vi "RampVoltagewithDDSV14.vi"() -> ()   [LabVIEW 2016]
uses:
  <vilib>/DAQmx/write.llb/DAQmx Write (Digital 1D Wfm NChan NSamp).vi
  <vilib>/DAQmx/write.llb/DAQmx Write (Analog 2D DBL NChan NSamp).vi
  <vilib>/DAQmx/create/channels.llb/DAQmx Create Channel (AO-Voltage-Basic).vi
  <vilib>/DAQmx/create/channels.llb/DAQmx Create Channel (DO-Digital Output).vi
  <vilib>/DAQmx/configure/timing.llb/DAQmx Timing (Sample Clock).vi
  <vilib>/DAQmx/configure/trigger.llb/DAQmx Start Trigger (Digital Edge).vi
  <vilib>/Waveform/DWDTOps.llb/DWDT Boolean Array to Digital.vi
  <vilib>/Waveform/DWDTOps.llb/DWDT Uncompress Digital.vi
  <vilib>/DAQmx/miscellaneous.llb/DAQmx Fill In Error Info.vi
  <vilib>/Waveform/DTblOps.llb/DTbl Digital to Analog.vi
  <resource>/objmgr/daqmx.rc
  <vilib>/Utility/file.llb/Write Delimited Spreadsheet (DBL).vi
panel:
  out "ao3 Samples":i32=2001
  out "ao2 Samples":i32=2001
  in  "ao3  File Path":path
  in  "ao2  File Path":path
  in  "Phase Lock Switch\n(TTL High - Lock Off)":bool
  in  "Phase Lock Switch (Port 0 Line 1)":tag="Dev2/port0/line1"
  out "Digital Output":cluster{i32, dbl, dbl[][]}(graph)={0, 1e-05, [[0.0, 0.0, 0.0, 0.0, 0.0, 0.0, 0.0, 0.0, 0.0, 0.0, 0.0, 0.0, 0.0, 0.0, 0.0, 0.0, 0.0, 0.0, 0.0, 0.0, 0.0, 0.0, 0.0, 0.0, 0.0, 0.0, 0.0, 0.0, 0.0, 0.0, 0.0, 0.0, 0.0, 0.0, 0.0, 0.0, 0.0, 0.0, 0.0, 0.0, 0.0, 0.0, 0.0, 0.0, 0.0, 0.0, 0.0, 0.0, 0.0, 0.0, 0.0, 0.0, 0.0, 0.0, 0.0, 0.0, 0.0, 0.0, 0.0, 0.0, 0.0, 0.0, 0.0, 0.0, 0.0, 0.0, 0.0, 0.0, 0.0, 0.0, 0.0, 0.0, 0.0, 0.0, 0.0, 0.0, 0.0, 0.0, 0.0, 0.0, 0.0, 0.0, 0.0, 0.0, 0.0, 0.0, 0.0, 0.0, 0.0, 0.0, 0.0, 0.0, 0.0, 0.0, 0.0, 0.0, 0.0, 0.0, 0.0, 0.0, 0.0, 0.0, 0.0, 0.0, 0.0, 0.0, 0.0, 0.0, 0.0, 0.0, 0.0, 0.0, 0.0, 0.0, 0.0, 0.0, 0.0, 0.0, 0.0, 0.0, 0.0, 0.0, 0.0, 5.0, 5.0, 5.0, 5.0, 5.0, 5.0, 5.0, 5.0, 5.0, 5.0, 5.0, 5.0, 5.0, 5.0, 5.0, 5.0, 5.0, 5.0, 5.0, 5.0, 5.0, 5.0, 5.0, 5.0, 5.0, 5.0, 5.0, 5.0, 5.0, 5.0, 5.0, 5.0, 5.0, 5.0, 5.0, 5.0, 5.0, 5.0, 5.0, 5.0, 5.0, 5.0, 5.0, 5.0, 5.0, 5.0, 5.0, 5.0, 5.0, 5.0, 5.0, 5.0, 5.0, 5.0, 5.0, 5.0, 5.0, 5.0, 5.0, 5.0, 5.0, 5.0, 5.0, 5.0, 5.0, 5.0, 5.0, 5.0, 5.0, 5.0, 5.0, 5.0, 5.0, 5.0, 5.0, 5.0, 5.0, 5.0, 5.0, 5.0, 5.0, 5.0, 5.0, 5.0, 5.0, 5.0, 5.0, 5.0, 5.0, 5.0, 5.0, 5.0, 5.0, 5.0, 5.0, 5.0, 5.0, 5.0, 5.0, 5.0, 5.0, 5.0, 5.0, 5.0, 5.0, 5.0, 5.0, 5.0, 5.0, 5.0, 5.0, 5.0, 5.0, 5.0, 5.0, 5.0, 5.0, 5.0, 5.0, 5.0, 5.0, 5.0, 5.0, 5.0, 5.0, 5.0, 5.0, 5.0, 5.0, 5.0, 5.0, 5.0, 5.0, 5.0, 5.0, 5.0, 5.0, 5.0, 5.0, 5.0, 5.0, 5.0, 5.0, 5.0, 5.0, 5.0, 5.0, 5.0, 5.0, 5.0, 5.0, 5.0, 5.0, 5.0, 5.0, 5.0, 5.0, 5.0, 5.0, 5.0, 5.0, 5.0, 5.0, 5.0, 5.0, 5.0, 5.0, 5.0, 5.0, 5.0, 5.0, 5.0, 5.0, 5.0, 5.0, 5.0, 5.0, 5.0, 5.0, 5.0, 5.0, 5.0, 5.0, 5.0, 5.0, 5.0, 5.0, 5.0, 5.0, 5.0, 5.0, 5.0, 5.0, 5.0, 5.0, 5.0, 5.0, 5.0, 5.0, 5.0, 5.0, 5.0, 5.0, 5.0, 5.0, 5.0, 5.0, 5.0, 5.0, 5.0, 5.0, 5.0, 5.0, 5.0, 5.0, 5.0, 5.0, 5.0, 5.0, 5.0, 5.0, 5.0, 5.0, 5.0, 5.0, 5.0, 5.0, 5.0, 5.0, 5.0, 5.0, 5.0, 5.0, 5.0, 5.0, 5.0, 5.0, 5.0, 5.0, 5.0, 5.0, 5.0, 5.0, 5.0, 5.0, 5.0, 5.0, 5.0, 5.0, 5.0, 5.0, 5.0, 5.0, 5.0, 5.0, 5.0, 5.0, 5.0, 5.0, 5.0, 5.0, 5.0, 5.0, 5.0, 5.0, 5.0, 5.0, 5.0, 5.0, 5.0, 5.0, 5.0, 5.0, 5.0, 5.0, 5.0, 5.0, 5.0, 5.0, 5.0, 5.0, 5.0, 5.0, 5.0, 5.0, 5.0, 5.0, 5.0, 5.0, 5.0, 5.0, 5.0, 5.0, 5.0, 5.0, 5.0, 5.0, 5.0, 5.0, 5.0, 5.0, 5.0, 5.0, 5.0, 5.0, 5.0, 5.0, 5.0, 5.0, 5.0, 5.0, 5.0, 5.0, 5.0, 5.0, 5.0, 5.0, 5.0, 5.0, 5.0, 5.0, 5.0, 5.0, 5.0, 5.0, 5.0, 5.0, 5.0, 5.0, 5.0, 5.0, 5.0, 5.0, 5.0, 5.0, 5.0, 5.0, 5.0, 5.0, 5.0, 5.0, 5.0, 5.0, 5.0, 5.0, 5.0, 5.0, 5.0, 5.0, 5.0, 5.0, 5.0, 5.0, 5.0, 5.0, 5.0, 5.0, 5.0, 5.0, 5.0, 5.0, 5.0, 5.0, 5.0, 5.0, 5.0, 5.0, 5.0, 5.0, 5.0, 5.0, 5.0, 5.0, 5.0, 5.0, 5.0, 5.0, 5.0, 5.0, 5.0, 5.0, 5.0, 5.0, 5.0, 5.0, 5.0, 5.0, 5.0, 5.0, 5.0, 5.0, 5.0, 5.0, 5.0, 5.0, 5.0, 5.0, 5.0, 5.0, 5.0, 0.0, 0.0, 0.0, 0.0, 0.0, 0.0, 0.0, 0.0, 0.0, 0.0, 0.0, 0.0, 0.0, 0.0, 0.0, 0.0, 0.0, 0.0, 0.0, 0.0, 0.0, 0.0, 0.0, 0.0, 0.0, 0.0, 0.0, 0.0, 0.0, 0.0, 0.0, 0.0, 0.0, 0.0, 0.0, 0.0, 0.0, 0.0, 0.0, 0.0, 0.0, 0.0, 0.0, 0.0, 0.0, 0.0, 0.0, 0.0, 0.0, 0.0, 0.0, 0.0, 0.0, 0.0, 0.0, 0.0, 0.0, 0.0, 0.0, 0.0, 0.0, 0.0, 0.0, 0.0, 0.0, 0.0, 0.0, 0.0, 0.0, 0.0, 0.0, 0.0, 0.0, 0.0, 0.0, 0.0, 0.0, 0.0, 0.0, 0.0, 0.0, 0.0, 0.0, 0.0, 0.0, 0.0, 0.0, 0.0, 0.0, 0.0, 0.0, 0.0, 0.0, 0.0, 0.0, 0.0, 0.0, 0.0, 0.0, 0.0, 0.0, 0.0, 0.0, 0.0, 0.0, 0.0, 0.0, 0.0, 0.0, 0.0, 0.0, 0.0, 0.0, 0.0, 0.0, 0.0, 0.0, 0.0, 0.0, 0.0, 0.0, 0.0, 0.0, 0.0, 0.0, 0.0, 0.0, 0.0, 0.0, 0.0, 0.0, 0.0, 0.0, 0.0, 0.0, 0.0, 0.0, 0.0, 0.0, 0.0, 0.0, 0.0, 0.0, 0.0, 0.0, 0.0, 0.0, 0.0, 0.0, 0.0, 0.0, 0.0, 0.0, 0.0, 0.0, 0.0, 0.0, 0.0, 0.0, 0.0, 0.0, 0.0, 0.0, 0.0, 0.0, 0.0, 0.0, 0.0, 0.0, 0.0, 0.0, 0.0, 0.0, 0.0, 0.0, 0.0, 0.0, 0.0, 0.0, 0.0, 0.0, 0.0, 0.0, 0.0, 0.0, 0.0, 0.0, 0.0, 0.0, 0.0, 0.0, 0.0, 0.0, 0.0, 0.0, 0.0, 0.0, 0.0, 0.0, 0.0, 0.0, 0.0, 0.0, 0.0, 0.0, 0.0, 0.0, 0.0, 0.0, 0.0, 0.0, 0.0, 0.0, 0.0, 0.0, 0.0, 0.0, 0.0, 0.0, 0.0, 0.0, 0.0, 0.0, 0.0, 0.0, 0.0, 0.0, 0.0, 0.0, 0.0, 0.0, 0.0, 0.0, 0.0, 0.0, 0.0, 0.0, 0.0, 0.0, 0.0, 0.0, 0.0, 0.0, 0.0, 0.0, 0.0, 0.0, 0.0, 0.0, 0.0, 0.0, 0.0, 0.0, 0.0, 0.0, 0.0, 0.0, 0.0, 0.0, 0.0, 0.0, 0.0, 0.0, 0.0, 0.0, 0.0, 0.0, 0.0, 0.0, 0.0, 0.0, 0.0, 0.0, 0.0, 0.0, 0.0, 0.0, 0.0], [0.0, 0.0, 0.0, 0.0, 0.0, 0.0, 0.0, 0.0, 0.0, 0.0, 0.0, 0.0, 0.0, 0.0, 0.0, 0.0, 0.0, 0.0, 0.0, 0.0, 0.0, 0.0, 0.0, 0.0, 0.0, 0.0, 0.0, 0.0, 0.0, 0.0, 0.0, 0.0, 0.0, 0.0, 0.0, 0.0, 0.0, 0.0, 0.0, 0.0, 0.0, 0.0, 0.0, 0.0, 0.0, 0.0, 0.0, 0.0, 0.0, 0.0, 0.0, 0.0, 0.0, 0.0, 0.0, 0.0, 0.0, 0.0, 0.0, 0.0, 0.0, 0.0, 0.0, 0.0, 0.0, 0.0, 0.0, 0.0, 0.0, 0.0, 0.0, 0.0, 0.0, 0.0, 0.0, 0.0, 0.0, 0.0, 0.0, 0.0, 0.0, 0.0, 0.0, 0.0, 0.0, 0.0, 0.0, 0.0, 0.0, 0.0, 0.0, 0.0, 0.0, 0.0, 0.0, 0.0, 0.0, 0.0, 0.0, 0.0, 0.0, 0.0, 0.0, 0.0, 0.0, 0.0, 0.0, 0.0, 0.0, 0.0, 0.0, 0.0, 0.0, 0.0, 0.0, 0.0, 0.0, 0.0, 0.0, 0.0, 0.0, 0.0, 0.0, 0.0, 0.0, 0.0, 0.0, 0.0, 0.0, 0.0, 0.0, 0.0, 0.0, 0.0, 0.0, 0.0, 0.0, 0.0, 0.0, 0.0, 0.0, 0.0, 0.0, 0.0, 0.0, 0.0, 0.0, 0.0, 0.0, 0.0, 0.0, 0.0, 0.0, 0.0, 0.0, 0.0, 0.0, 0.0, 0.0, 0.0, 0.0, 0.0, 0.0, 0.0, 0.0, 0.0, 0.0, 0.0, 0.0, 0.0, 0.0, 0.0, 0.0, 0.0, 0.0, 0.0, 0.0, 0.0, 0.0, 0.0, 0.0, 0.0, 0.0, 0.0, 0.0, 0.0, 0.0, 0.0, 0.0, 0.0, 0.0, 0.0, 0.0, 0.0, 0.0, 0.0, 0.0, 0.0, 0.0, 0.0, 0.0, 0.0, 0.0, 0.0, 0.0, 0.0, 0.0, 0.0, 0.0, 0.0, 0.0, 0.0, 0.0, 0.0, 0.0, 0.0, 0.0, 0.0, 0.0, 0.0, 0.0, 0.0, 0.0, 0.0, 0.0, 0.0, 0.0, 0.0, 0.0, 0.0, 0.0, 0.0, 0.0, 0.0, 0.0, 0.0, 0.0, 0.0, 0.0, 0.0, 0.0, 0.0, 0.0, 0.0, 0.0, 0.0, 0.0, 0.0, 0.0, 0.0, 0.0, 0.0, 0.0, 0.0, 0.0, 0.0, 0.0, 0.0, 0.0, 0.0, 0.0, 0.0, 0.0, 0.0, 0.0, 0.0, 0.0, 0.0, 0.0, 0.0, 0.0, 0.0, 0.0, 0.0, 0.0, 0.0, 0.0, 0.0, 0.0, 0.0, 0.0, 0.0, 0.0, 0.0, 0.0, 0.0, 0.0, 0.0, 0.0, 0.0, 0.0, 0.0, 0.0, 0.0, 0.0, 0.0, 0.0, 0.0, 0.0, 0.0, 0.0, 0.0, 0.0, 0.0, 0.0, 0.0, 0.0, 0.0, 0.0, 0.0, 0.0, 0.0, 0.0, 0.0, 0.0, 0.0, 0.0, 0.0, 0.0, 0.0, 0.0, 0.0, 0.0, 0.0, 0.0, 0.0, 0.0, 0.0, 0.0, 0.0, 0.0, 0.0, 0.0, 0.0, 0.0, 0.0, 0.0, 0.0, 0.0, 0.0, 0.0, 0.0, 0.0, 0.0, 0.0, 0.0, 0.0, 0.0, 0.0, 0.0, 0.0, 0.0, 0.0, 0.0, 0.0, 0.0, 0.0, 0.0, 0.0, 0.0, 0.0, 0.0, 0.0, 0.0, 0.0, 0.0, 0.0, 0.0, 0.0, 0.0, 0.0, 0.0, 0.0, 0.0, 0.0, 0.0, 0.0, 0.0, 0.0, 0.0, 0.0, 0.0, 0.0, 0.0, 0.0, 0.0, 0.0, 0.0, 0.0, 0.0, 0.0, 0.0, 0.0, 0.0, 0.0, 0.0, 0.0, 0.0, 0.0, 0.0, 0.0, 0.0, 0.0, 0.0, 0.0, 0.0, 0.0, 0.0, 0.0, 0.0, 0.0, 0.0, 0.0, 0.0, 0.0, 0.0, 0.0, 0.0, 0.0, 0.0, 0.0, 0.0, 0.0, 0.0, 0.0, 0.0, 0.0, 0.0, 0.0, 0.0, 0.0, 0.0, 0.0, 0.0, 0.0, 0.0, 0.0, 0.0, 0.0, 0.0, 0.0, 0.0, 0.0, 0.0, 0.0, 0.0, 0.0, 0.0, 0.0, 0.0, 0.0, 0.0, 0.0, 0.0, 0.0, 0.0, 0.0, 0.0, 0.0, 0.0, 0.0, 0.0, 0.0, 0.0, 0.0, 0.0, 0.0, 0.0, 0.0, 0.0, 0.0, 0.0, 0.0, 0.0, 0.0, 0.0, 0.0, 0.0, 0.0, 0.0, 0.0, 0.0, 0.0, 0.0, 0.0, 0.0, 0.0, 0.0, 0.0, 0.0, 0.0, 0.0, 0.0, 0.0, 0.0, 0.0, 0.0, 0.0, 0.0, 0.0, 0.0, 0.0, 0.0, 0.0, 0.0, 0.0, 0.0, 0.0, 0.0, 0.0, 0.0, 0.0, 0.0, 0.0, 0.0, 0.0, 0.0, 0.0, 0.0, 0.0, 0.0, 0.0, 0.0, 0.0, 0.0, 0.0, 0.0, 0.0, 0.0, 0.0, 0.0, 0.0, 0.0, 0.0, 0.0, 0.0, 0.0, 0.0, 0.0, 0.0, 0.0, 0.0, 0.0, 0.0, 0.0, 0.0, 0.0, 0.0, 0.0, 0.0, 0.0, 0.0, 0.0, 0.0, 0.0, 0.0, 0.0, 0.0, 0.0, 0.0, 0.0, 0.0, 0.0, 0.0, 0.0, 0.0, 0.0, 0.0, 0.0, 0.0, 0.0, 0.0, 0.0, 0.0, 0.0, 0.0, 0.0, 0.0, 0.0, 0.0, 0.0, 0.0, 0.0, 0.0, 0.0, 0.0, 0.0, 0.0, 0.0, 0.0, 0.0, 0.0, 0.0, 0.0, 0.0, 0.0, 0.0, 0.0, 0.0, 0.0, 0.0, 0.0, 0.0, 0.0, 0.0, 0.0, 0.0, 0.0, 0.0, 0.0, 0.0, 0.0, 0.0, 0.0, 0.0, 0.0, 0.0, 0.0, 0.0, 0.0, 0.0, 0.0, 0.0, 0.0, 0.0, 0.0, 0.0, 0.0, 0.0, 0.0, 0.0, 0.0, 0.0, 0.0, 0.0, 0.0, 0.0, 0.0, 0.0, 0.0, 0.0, 0.0, 0.0, 0.0, 0.0, 0.0, 0.0, 0.0, 0.0, 0.0, 0.0, 0.0, 0.0, 0.0, 0.0, 0.0, 0.0, 0.0, 0.0, 0.0, 0.0, 0.0, 0.0, 0.0, 0.0, 0.0, 0.0, 0.0, 0.0, 0.0, 0.0, 0.0, 0.0, 0.0, 0.0, 0.0, 0.0, 0.0, 0.0, 0.0, 0.0, 0.0, 0.0, 0.0, 0.0, 0.0, 0.0, 0.0, 0.0, 0.0, 0.0, 0.0, 0.0, 0.0, 0.0, 0.0, 0.0, 0.0, 0.0, 0.0, 0.0, 0.0, 0.0, 0.0, 0.0, 0.0, 0.0, 0.0, 0.0, 0.0, 0.0, 0.0, 0.0, 0.0, 0.0, 0.0, 0.0, 0.0, 0.0, 0.0, 0.0, 0.0, 0.0, 0.0, 0.0, 0.0, 0.0, 0.0, 0.0, 0.0, 0.0, 0.0, 0.0, 0.0, 0.0, 0.0, 0.0, 0.0, 0.0, 0.0, 0.0, 0.0, 0.0, 0.0, 0.0, 0.0, 0.0, 0.0, 0.0, 0.0, 0.0, 0.0, 0.0, 0.0, 0.0, 0.0, 0.0, 0.0, 0.0, 0.0, 0.0, 0.0, 0.0, 0.0, 0.0, 0.0, 0.0, 0.0, 0.0, 0.0, 0.0, 0.0, 0.0, 0.0, 0.0, 0.0, 0.0, 0.0, 0.0, 0.0, 0.0, 0.0, 0.0, 0.0, 0.0, 0.0, 0.0, 0.0, 0.0, 0.0, 0.0, 0.0, 0.0, 0.0, 0.0, 0.0, 0.0, 0.0, 0.0, 0.0, 0.0]]}
  out "Analog Outputs":cluster{i32, dbl, dbl[][]}(graph)={0, 4e-06, array4x2001[8004 elements]}
  in  "DDS Trigger (Port 0 Line 0)":tag="Dev2/port0/line0"
  in  "DDS trigger delay (ms)":dbl=0.23 step=0.01
  in  "error in 2":errorcluster caption="error in"
  in  "ao3 ramp amplitude (V)":dbl
  in  "ao2 ramp amplitude (V)":dbl
  in  "ao1 ramp amplitude (V)":dbl=0.04
  in  "SolsTiS 2 - Fast Piezo (ao3)":tag="Dev2/ao3"
  in  "SolsTiS 2 - Slow Piezo (ao2)":tag="Dev2/ao2"
  out "Generated Ramp Samples":i32=2001
  in  "Trigger delay NI (ms)":dbl=1.0
  in  "Trigger Input (PFI0)":tag="/Dev2/PFI0"
  in  "SolsTiS 1 - Fast Piezo (ao1)":tag="Dev2/ao1"
  in  "SolsTiS 1 - Slow Piezo (ao0)":tag="Dev2/ao0"
  in  "Plateau duration (ms)":dbl=2.0 step=0.01
  in  "Ramp duration (ms)":dbl=2.0 step=0.01
  in  "ao0 ramp amplitude (V)":dbl=0.09 step=0.001
  in  "error in":errorcluster
  # "MAGIS LASER SYSTEM\nChirp Control"
  # "Ramp Definition"
  # "Output Monitor"
  # "Channel Definition"
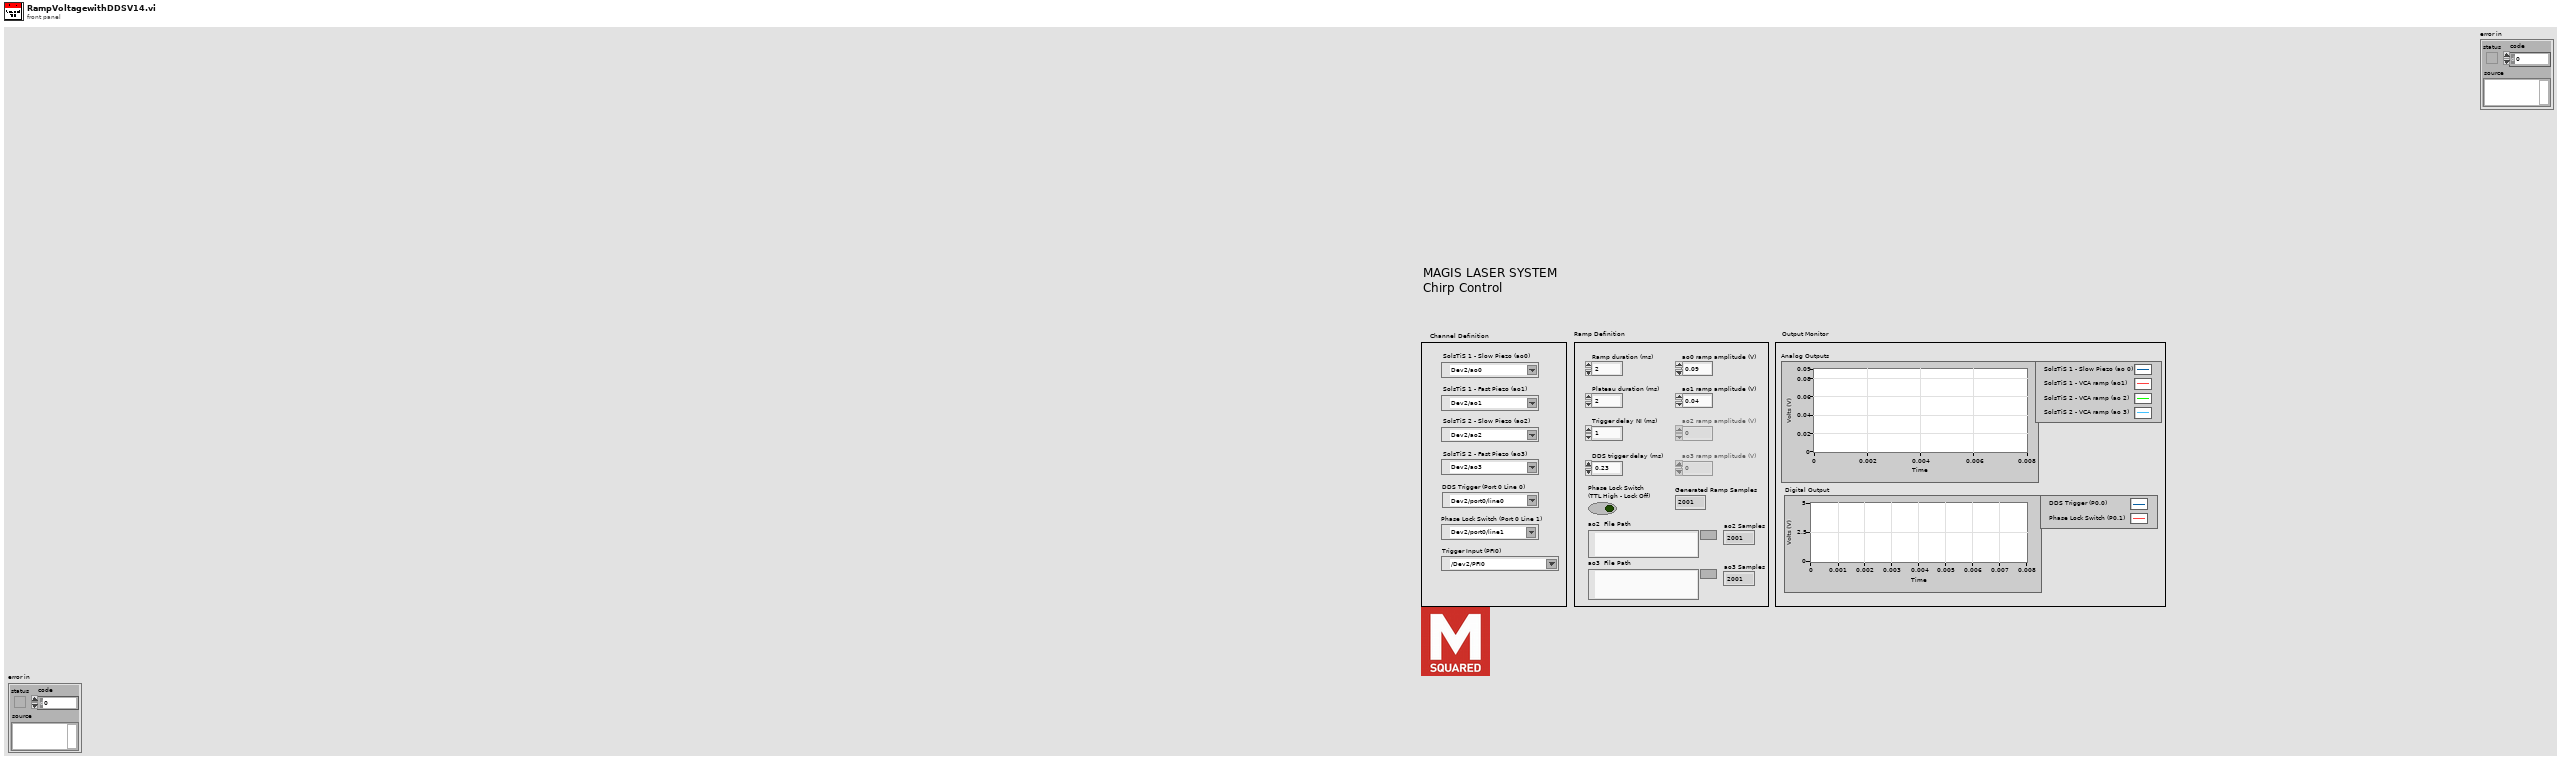
[diagram p1: front panel]
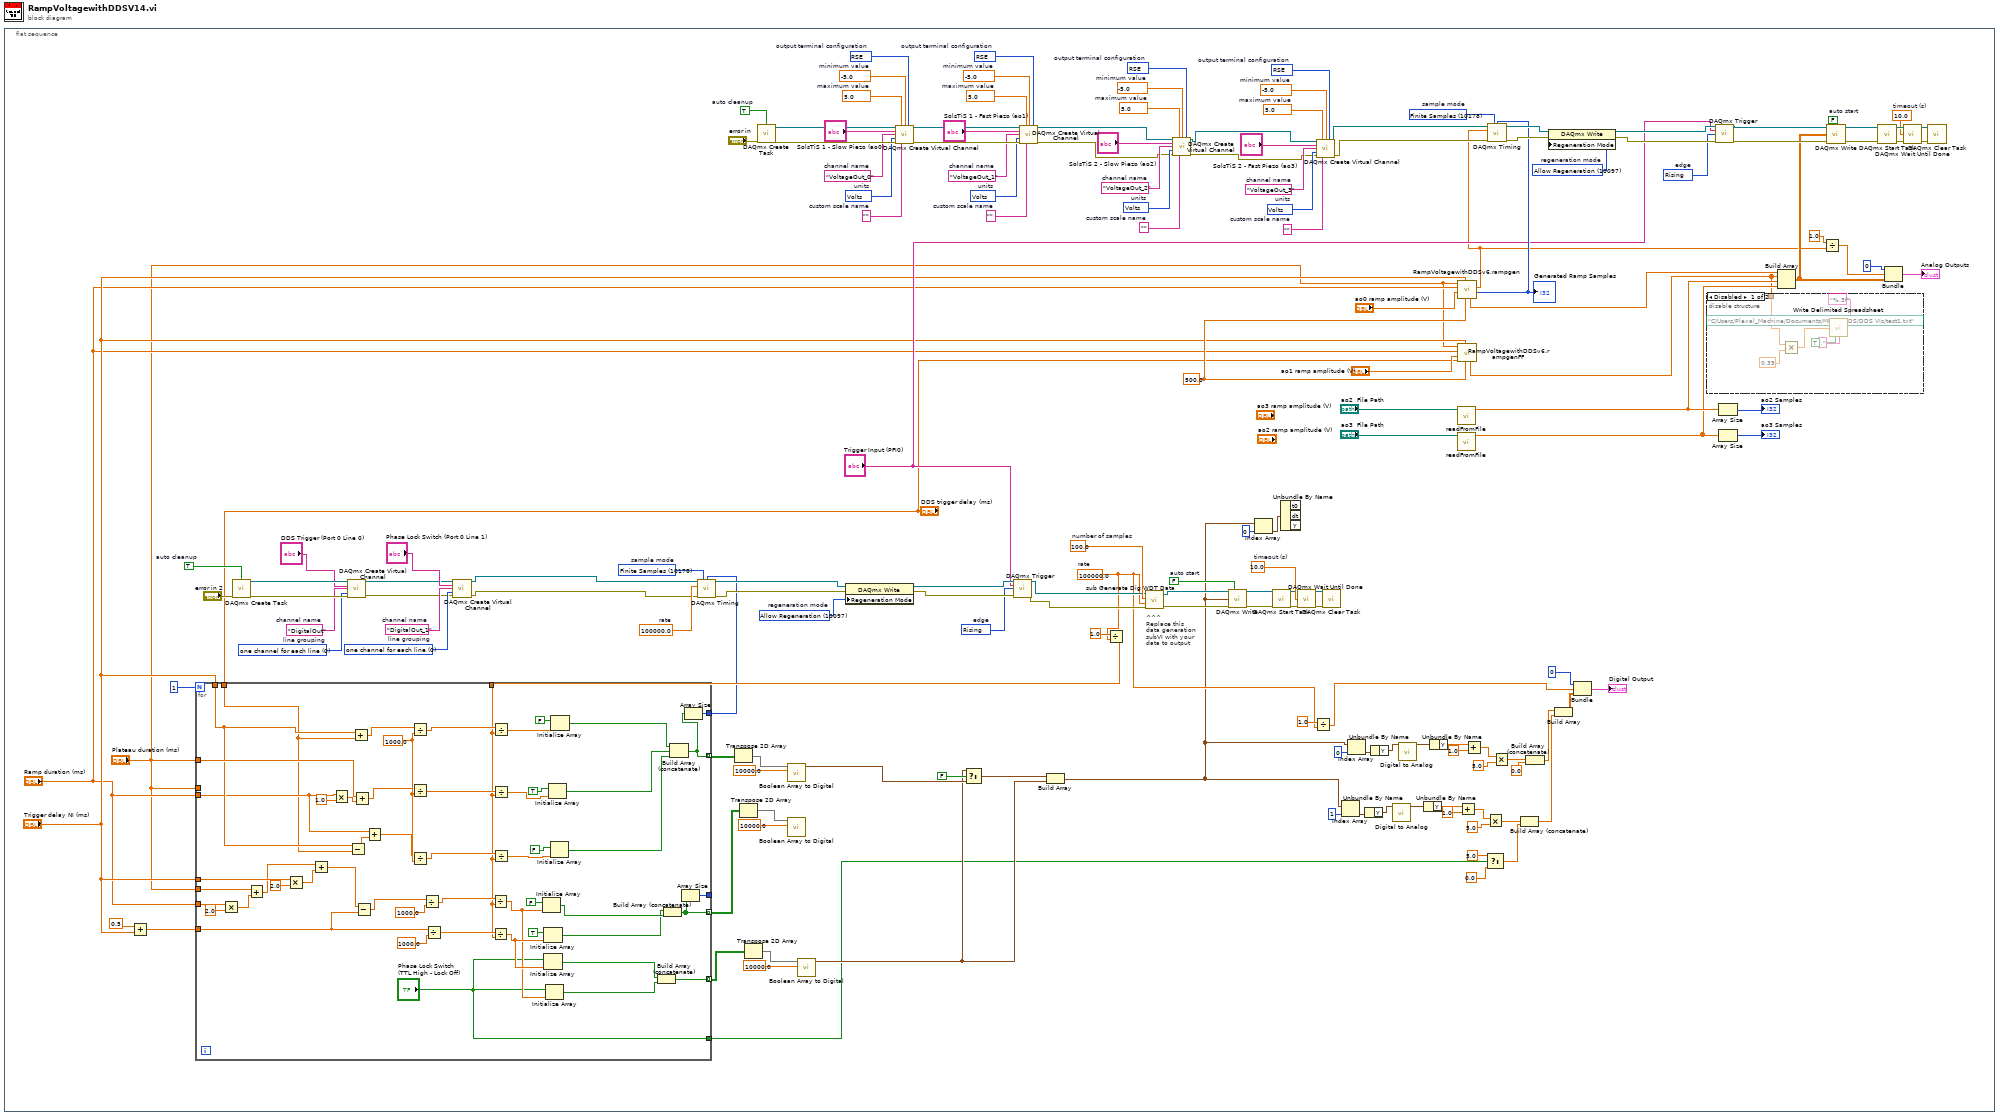
[diagram p0: block diagram]
diagram:
  n1 = flat-sequence {
    frame #0 {
      w46 = 0 items=["one channel for each line", "one channel for all lines"]  # line grouping
      w45 = "DigitalOut_1"  # channel name
      w108 = 500.0 ("No of samples in ramp (500 or less)")
      w80 = 10280 items=["Rising"=10280, "Falling"=10171]  # edge
      w82 = 10097 items=["Allow Regeneration"=10097, "Do Not Allow Regeneration"=10158]  # regeneration mode
      w85 = 10178 items=["Finite Samples"=10178, "Continuous Samples"=10123, "Hardware Timed Single Point"=12522]  # sample mode
      w86 = 100000.0  # rate
      w89 = 0 items=["one channel for each line", "one channel for all lines"]  # line grouping
      w88 = "DigitalOut"  # channel name
      w91 = TRUE  # auto cleanup
      w106 = 10.0  # timeout (s)
      w54 = 100000.0  # rate
      w99 = 100.0  # number of samples
      w96 = FALSE  # auto start
      w115 = 10083 items=["Default"=-1, "RSE"=10083, "Differential"=10106, "Pseudodifferential"=12529]  # output terminal configuration
      w116 = 10348 items=["Volts"=10348, "From Custom Scale"=10065]  # units
      w117 = "VoltageOut_3"  # channel name
      w118 = ""  # custom scale name
      w119 = -5.0  # minimum value
      w120 = 5.0  # maximum value
      w124 = 10083 items=["Default"=-1, "RSE"=10083, "Differential"=10106, "Pseudodifferential"=12529]  # output terminal configuration
      w125 = 10348 items=["Volts"=10348, "From Custom Scale"=10065]  # units
      w126 = "VoltageOut_2"  # channel name
      w127 = ""  # custom scale name
      w128 = -5.0  # minimum value
      w129 = 5.0  # maximum value
      w136 = 10280 items=["Rising"=10280, "Falling"=10171]  # edge
      w138 = 10097 items=["Allow Regeneration"=10097, "Do Not Allow Regeneration"=10158]  # regeneration mode
      w141 = 10178 items=["Finite Samples"=10178, "Continuous Samples"=10123, "Hardware Timed Single Point"=12522]  # sample mode
      w143 = 10083 items=["Default"=-1, "RSE"=10083, "Differential"=10106, "Pseudodifferential"=12529]  # output terminal configuration
      w144 = 10348 items=["Volts"=10348, "From Custom Scale"=10065]  # units
      w145 = "VoltageOut_1"  # channel name
      w146 = ""  # custom scale name
      w147 = -5.0  # minimum value
      w148 = 5.0  # maximum value
      w150 = 10083 items=["Default"=-1, "RSE"=10083, "Differential"=10106, "Pseudodifferential"=12529]  # output terminal configuration
      w151 = 10348 items=["Volts"=10348, "From Custom Scale"=10065]  # units
      w152 = "VoltageOut_0"  # channel name
      w154 = ""  # custom scale name
      w155 = -5.0  # minimum value
      w156 = 5.0  # maximum value
      w158 = TRUE  # auto cleanup
      w164 = 10.0  # timeout (s)
      w168 = FALSE  # auto start
      # "^^^\nReplace this\ndata generation\nsubVI with your\ndata to output"
      n2 = Add(x=0.5 ("DDS Trigger delay (ms)"), y="Trigger delay NI (ms)") -> (x+y=w40:dbl)
      n3 = call <vilib>:"DAQmx Create Task.vi"("auto cleanup"=w91, "error in"="error in 2") -> ("task out"=w90:refnum<k21>, "error out"=w92:errorcluster)  [unwired: 12 in]
      n4 = call-poly <vilib>:"DAQmx Create Virtual Channel.vi"("task in"=w90, "lines"="DDS Trigger (Port 0 Line 0)", "name to assign"=w88, "line grouping"=w89, "error in"=w92) -> ("task out"=w42:refnum<k21>, "error out"=w43:errorcluster)  [unwired: 9 in]
      n5 = call-poly <vilib>:"DAQmx Create Virtual Channel.vi"("task in"=w42, "lines"="Phase Lock Switch (Port 0 Line 1)", "name to assign"=w45, "line grouping"=w46, "error in"=w43) -> ("task out"=w18:refnum<k21>, "error out"=w17:errorcluster)  [unwired: 9 in]
      n6 = call <vilib>:"DAQmx Create Task.vi"("auto cleanup"=w158, "error in"="error in") -> ("task out"=w157:refnum<k21>, "error out"=w159:errorcluster)  [unwired: 12 in]
      n7 = call-poly <vilib>:"DAQmx Create Virtual Channel.vi"("task in"=w157, "maximum value"=w156, "minimum value"=w155, "output terminal configuration"=w150, "physical channels"="SolsTiS 1 - Slow Piezo (ao0)", "name to assign"=w152, "units"=w151, "error in"=w159, "custom scale name"=w154) -> ("task out"=w149:refnum<k21>, "error out"=w153:errorcluster)  [unwired: 5 in]
      n8 = call-poly <vilib>:"DAQmx Create Virtual Channel.vi"("task in"=w149, "maximum value"=w148, "minimum value"=w147, "output terminal configuration"=w143, "physical channels"="SolsTiS 1 - Fast Piezo (ao1)", "name to assign"=w145, "units"=w144, "error in"=w153, "custom scale name"=w146) -> ("task out"=w122:refnum<k21>, "error out"=w121:errorcluster)  [unwired: 5 in]
      n9 = Divide(x=1.0, y=w54) -> (x/y=w76:dbl)
      n10 = for {
        N: 1 -> [_]
        tunnel: w76 -> [w202]
        tunnel: [w217] -> w73 mode=indexing
        tunnel: [w216] -> w72
        tunnel: "Plateau duration (ms)" -> [_]
        tunnel: "Trigger delay NI (ms)" -> [w181]
        tunnel: w40 -> [w208]
        tunnel: "Ramp duration (ms)" -> [w212]
        tunnel: "Plateau duration (ms)" -> [w209]
        tunnel: [w199] -> _
        tunnel: "Trigger delay NI (ms)" -> [w196]
        tunnel: [w193] -> w36 mode=indexing
        tunnel: [w189] -> w33 mode=indexing
        tunnel: "Ramp duration (ms)" -> [w179]
        tunnel: "Plateau duration (ms)" -> [w183]
        tunnel: ["Phase Lock Switch\n(TTL High - Lock Off)"] -> w13
        tunnel: "DDS trigger delay (ms)" -> [w176]
        w227 = 1000.0
        n11 = Multiply(x=w212, y=2.0) -> (x*y=w210:dbl)
        n12 = Add(x=w209, y=w210) -> (x+y=w195:dbl)
        n13 = Multiply(x=w196, y=2.0) -> (x*y=w197:dbl)
        n14 = Add(x=w195, y=w197) -> (x+y=w194:dbl)
        n15 = Multiply(x=w179, y=1.0) -> (x*y=w184:dbl)
        n16 = Subtract(x=w181, y=w176) -> (x-y=w178:dbl)
        n17 = Add(x=w181, y=w176) -> (x+y=w215:dbl)
        n18 = Add(x=w183, y=w184) -> (x+y=w182:dbl)
        n19 = Subtract(x=w194, y=w208) -> (x-y=w205:dbl)
        n20 = Add(x=w179, y=w178) -> (x+y=w177:dbl)
        n21 = Divide(x=w215, y=w227) -> (x/y=w226:dbl)
        n22 = Divide(x=w182, y=w227) -> (x/y=w225:dbl)
        n23 = Divide(x=w177, y=w227) -> (x/y=w224:dbl)
        n24 = Divide(x=w205, y=1000.0) -> (x/y=w204:dbl)
        n25 = Divide(x=w208, y=1000.0) -> (x/y=w203:dbl)
        n26 = Divide(x=w204, y=w202) -> (x/y=w188:dbl)
        n27 = Divide(x=w203, y=w202) -> (x/y=w192:dbl)
        n28 = Divide(x=w226, y=w202) -> (x/y=w221:dbl)
        n29 = Divide(x=w225, y=w202) -> (x/y=w220:dbl)
        n30 = Divide(x=w224, y=w202) -> (x/y=w219:dbl)
        n31 = Initialize Array(FALSE, w188) -> (w201:bool[])
        n32 = Initialize Array(TRUE, w192) -> (w200:bool[])
        n33 = Initialize Array("Phase Lock Switch\n(TTL High - Lock Off)", w192) -> (w191:bool[])
        n34 = Initialize Array("Phase Lock Switch\n(TTL High - Lock Off)", w188) -> (w190:bool[])
        n35 = Initialize Array(TRUE, w220) -> (w187:bool[])
        n36 = Initialize Array(FALSE, w219) -> (w186:bool[])
        n37 = Initialize Array(FALSE, w221) -> (w218:bool[])
        n38 = Build Array (concatenate)(w191, w190) -> (w189:bool[])
        n39 = Build Array (concatenate)(w200, w201) -> (w193:bool[])
        n40 = Build Array (concatenate)(w218, w187, w186) -> (w217:bool[])
        n41 = Array Size(array=w193) -> (size(s)=w199:i32)
        n42 = Array Size(array=w217) -> (size(s)=w216:i32)
      }
      n43 = call-poly <vilib>:"DAQmx Timing.vi"("task/channels in"=w18, "sample mode"=w85, "samples per channel"=w72, "rate"=w86, "error in"=w17) -> ("task out"=w84:refnum<k21>, "error out"=w87:errorcluster)  [unwired: 9 in]
      n44 = Transpose 2D Array(2D array=w73) -> (transposed array=w74:bool[][])
      n45 = Transpose 2D Array(2D array=w36) -> (transposed array=w37:bool[][])
      n46 = Transpose 2D Array(2D array=w33) -> (transposed array=w34:bool[][])
      n47 = call-poly <vilib>:"Boolean Array to Digital.vi"("sample rate"=10000.0, "boolean array"=w74) -> ("digital waveform"=w22:digitalwaveform)  [unwired: 8 in, 1 out]
      n48 = call-poly <vilib>:"Boolean Array to Digital.vi"("sample rate"=10000.0, "boolean array"=w37) -> ()  [unwired: 8 in, 2 out]
      n49 = call-poly <vilib>:"Boolean Array to Digital.vi"("sample rate"=10000.0, "boolean array"=w34) -> ("digital waveform"=w14:digitalwaveform)  [unwired: 8 in, 1 out]
      n50 = property class="DAQmx Write"(reference=w84, error in=w87, "Regeneration Mode"=w82) -> (reference out=w81:refnum<k21>, error out=w83:errorcluster)
      n51 = Select(t=w14, s=FALSE ("Constant PO.0?"), f=w22) -> (s? t:f=w20:digitalwaveform)
      n52 = call-poly <vilib>:"DAQmx Trigger.vi"("task/channels in"=w81, "source"="Trigger Input (PFI0)", "edge"=w80, "error in"=w83) -> ("task out"=w79:refnum<k21>, "error out"=w78:errorcluster)  [unwired: 10 in]
      n53 = Build Array(w20, w14) -> (w19:digitalwaveform[])
      n54 = call <vilib>:"sub Generate Dig WDT Data.vi"("task in"=w79, "number of samples"=w99, "update rate"=w54, "error in"=w78) -> ("task out"=w98:refnum<k21>, "error out"=w97:errorcluster)  [unwired: 1 in, 1 out]
      n55 = call-poly <vilib>:"DAQmx Create Virtual Channel.vi"("task in"=w122, "maximum value"=w129, "minimum value"=w128, "output terminal configuration"=w124, "physical channels"="SolsTiS 2 - Slow Piezo (ao2)", "name to assign"=w126, "units"=w125, "error in"=w121, "custom scale name"=w127) -> ("task out"=w113:refnum<k21>, "error out"=w112:errorcluster)  [unwired: 5 in]
      n56 = call-poly <vilib>:"DAQmx Write.vi"("task/channels in"=w98, "auto start"=w96, "data"=w19, "error in"=w97) -> ("task out"=w103:refnum<k21>, "error out"=w104:errorcluster)  [unwired: 9 in, 1 out]
      n57 = Index Array(array=w19, index=0) -> (element=w94:digitalwaveform)
      n58 = call <vilib>:"DAQmx Start Task.vi"("task/channels in"=w103, "error in"=w104) -> ("task out"=w100:refnum<k21>, "error out"=w101:errorcluster)  [unwired: 12 in]
      n59 = Unbundle By Name(w94) -> ()  [unwired: 3 out]
      n60 = call <vilib>:"DAQmx Wait Until Done.vi"("task/channels in"=w100, "timeout (sec)"=w106, "error in"=w101) -> ("task out"=w105:refnum<k21>, "error out"=w102:errorcluster)  [unwired: 11 in]
      n61 = Divide(x=1.0, y=w54) -> (x/y=w53:dbl)
      n62 = call-poly <vilib>:"DAQmx Create Virtual Channel.vi"("task in"=w113, "maximum value"=w120, "minimum value"=w119, "output terminal configuration"=w115, "physical channels"="SolsTiS 2 - Fast Piezo (ao3)", "name to assign"=w117, "units"=w116, "error in"=w112, "custom scale name"=w118) -> ("task out"=w110:refnum<k21>, "error out"=w111:errorcluster)  [unwired: 5 in]
      n63 = call <vilib>:"DAQmx Clear Task.vi"("task in"=w105, "error in"=w102) -> ()  [unwired: 13 in, 1 out]
      n64 = Index Array(array=w19, index=1) -> (element=w31:digitalwaveform)
      n65 = Index Array(array=w19, index=0) -> (element=w64:digitalwaveform)
      n66 = Unbundle By Name(w31) -> ("Y"=w30:digitaldata)
      n67 = Unbundle By Name(w64) -> ("Y"=w63:digitaldata)
      n68 = call-poly <vilib>:"Digital to Analog.vi"("digital table"=w30) -> ("analog waveform"=w29:waveform(dbl))  [unwired: 7 in, 3 out]
      n69 = call-poly <vilib>:"Digital to Analog.vi"("digital table"=w63) -> ("analog waveform"=w62:waveform(dbl))  [unwired: 7 in, 3 out]
      n70 = Unbundle By Name(w29) -> ("Y"=w27:dbl[])
      n71 = Unbundle By Name(w62) -> ("Y"=w51:dbl[])
      n72 = call "readFromFile.vi"("file path (dialog if empty)"="ao2  File Path") -> ("data"=w8:dbl[])  [unwired: 10 in]
      n73 = call "readFromFile.vi"("file path (dialog if empty)"="ao3  File Path") -> ("data"=w7:dbl[])  [unwired: 10 in]
      n74 = call "RampVoltagewithDDSv6,rampgen.vi"("No of samples in ramp"=w108, "Trigger delay NI (ms)"="Trigger delay NI (ms)", "Ramp Amplitude (V)}"="ao0 ramp amplitude (V)", "Ramp duration (ms)"="Ramp duration (ms)", "Plateau duration (ms)"="Plateau duration (ms)") -> ("Numeric 2"=w132:i32, "Numeric"=w57:dbl, "Array"=w109:dbl[])  [unwired: 3 in, 1 out]
      "Generated Ramp Samples" <- w132
      n75 = call "RampVoltagewithDDSv6,rampgenFF.vi"("No of samples in ramp"=w108, "Trigger delay NI (ms)"="Trigger delay NI (ms)", "DDS Trigger Delay (ms)"="DDS trigger delay (ms)", "Ramp Amplitude (V)}"="ao1 ramp amplitude (V)", "Ramp duration (ms)"="Ramp duration (ms)", "Plateau duration (ms)"="Plateau duration (ms)") -> ("Array"=w1:dbl[])  [unwired: 2 in, 3 out]
      n76 = Add(x=w27, y=1.0) -> (x+y=w26:dbl[])
      n77 = Add(x=w51, y=1.0) -> (x+y=w50:dbl[])
      n78 = Select(t=5.0, s=w13, f=0.0 ("y")) -> (s? t:f=w10:dbl)
      n79 = Multiply(x=w26, y=5.0) -> (x*y=w24:dbl[])
      n80 = call-poly <vilib>:"DAQmx Timing.vi"("task/channels in"=w110, "sample mode"=w141, "samples per channel"=w132, "rate"=w57, "error in"=w111) -> ("task out"=w140:refnum<k21>, "error out"=w142:errorcluster)  [unwired: 9 in]
      n81 = Multiply(x=w50, y=5.0) -> (x*y=w48:dbl[])
      n82 = Build Array (concatenate)(w24, w10) -> (w23:dbl[])
      n83 = Build Array (concatenate)(w48, 0.0 ("y")) -> (w47:dbl[])
      n84 = property class="DAQmx Write"(reference=w140, error in=w142, "Regeneration Mode"=w138) -> (reference out=w137:refnum<k21>, error out=w139:errorcluster)
      n85 = Build Array(w47, w23) -> (w59:dbl[][])
      n86 = Bundle(0, w53, w59) -> (→"Digital Output":cluster{i32, dbl, dbl[][]})  [unwired: 1 in]
      n87 = disable-structure shown="Disabled" {
        disable-tunnel: w1 -> [w171 _]
        frame Disabled {
          n88 = Multiply(x=w171, y=0.35 ("x")) -> (x*y=w169:dbl[])
          n89 = call-poly <vilib>:"Write Delimited Spreadsheet.vi"("file path (dialog if empty)"=path "C:/Users/Plexal_Machine/Documents/MM2toDDS/DDS VIs/test1.txt", "format (%.3f)"="%.3f", "1D data"=w169, "transpose? (no:F)"=TRUE, "delimiter (\\t)"="," ("delimiter (\\t)")) -> ()  [unwired: 9 in, 2 out]
        }
        frame Enabled {
        }
      }
      n90 = call-poly <vilib>:"DAQmx Trigger.vi"("task/channels in"=w137, "source"="Trigger Input (PFI0)", "edge"=w136, "error in"=w139) -> ("task out"=w134:refnum<k21>, "error out"=w133:errorcluster)  [unwired: 10 in]
      n91 = Array Size(array=w8) -> (size(s)=→"ao2 Samples":i32)
      n92 = Array Size(array=w7) -> (size(s)=→"ao3 Samples":i32)
      n93 = Build Array(w109, w1, w8, w7) -> (w68:dbl[][])
      n94 = Divide(x=1.0, y=w57) -> (x/y=w56:dbl)
      n95 = call-poly <vilib>:"DAQmx Write.vi"("task/channels in"=w134, "auto start"=w168, "data"=w68, "error in"=w133) -> ("task out"=w163:refnum<k21>, "error out"=w162:errorcluster)  [unwired: 9 in, 1 out]
      n96 = call <vilib>:"DAQmx Start Task.vi"("task/channels in"=w163, "error in"=w162) -> ("task out"=w167:refnum<k21>, "error out"=w166:errorcluster)  [unwired: 12 in]
      n97 = Bundle(0, w56, w68) -> (→"Analog Outputs":cluster{i32, dbl, dbl[][]})  [unwired: 1 in]
      n98 = call <vilib>:"DAQmx Wait Until Done.vi"("task/channels in"=w167, "timeout (sec)"=w164, "error in"=w166) -> ("task out"=w161:refnum<k21>, "error out"=w165:errorcluster)  [unwired: 11 in]
      n99 = call <vilib>:"DAQmx Clear Task.vi"("task in"=w161, "error in"=w165) -> ()  [unwired: 13 in, 1 out]
    }
  }
